vi "__anritsu_collect_data.vi"(1 "Points to read":i32) -> (0 "Data out":dbl[](array[numeric]))   [LabVIEW 2013]
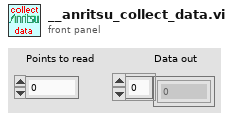
[diagram p1: front panel]
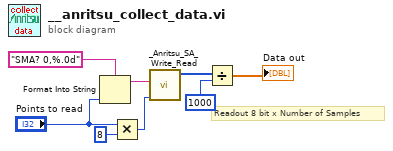
[diagram p0: block diagram]
diagram:
  # "Readout 8 bit x Number of Samples"
  n1 = Format Into String(format string="SMA? 0,%.0d" ("Comand"), "Points to read") -> (resulting string=w7:string)  [unwired: 2 in, 1 out]
  n2 = Multiply(x="Points to read", y=8) -> (x*y=w5:i32)
  n3 = call "_Anritsu_SA_Write_Read.vi"("bytes to read"=w5, "Comand"=w7) -> ("Data out"=w2:i32[])  [unwired: 4 in, 1 out]
  n4 = Divide(x=w2, y=1000) -> (x/y=→"Data out":dbl[])
